vi "CodigoLabView 4_1 2024.vi"() -> (11 "Releb 2":bool)   [LabVIEW 2024]
uses:
  <vilib>/addons/_office/NI_ReportGenerationToolkit.lvlib
  <vilib>/addons/_office/excel.llb/Excel Easy Table (str).vi
  <vilib>/Utility/NIReport.llb/NI_report.lvclass
  <vilib>/Utility/NIReport.llb/Report Type.ctl
  <vilib>/Utility/NIReport.llb/NI_ReportGenerationCore.lvlib
  <vilib>/Utility/NIReport.llb/Excel/NI_Excel.lvclass
  <vilib>/Instr/_visa.llb/VISA Configure Serial Port (Instr).vi
panel:
  out "RI 4":bool
  out "RI 3":bool
  out "RI 2":bool
  out "RS 4":bool
  out "RS 3":bool
  out "RS 2":bool
  out "RS 1":bool
  out "RI 1":bool
  out "errorout":errorcluster
  out "Vrno":refnum<visa-resource-name>
  out "Texto":path=path "C:/Users/Lucas Navarro/Desktop/Ruka/ME2/pf/Jamon.txt"
  out "Historial Tensión de Línea":dbl[](graph)
  out "Historial Tomacorriente 4":dbl[](graph)
  out "Historial Tomacorriente 3":dbl[](graph)
  out "Historial Tomacorriente 2":dbl[](graph)
  out "Historial Tomacorriente 1":dbl[](graph)
  in  "?":bool
  in  "RUTA DE REGISTRO":path
  out "NP4":dbl(knob) scale=0.0..100.0
  out "NP3":dbl(knob) scale=0.0..100.0
  out "NP2":dbl(knob) scale=0.0..100.0
  out "R ON 4":bool
  out "R ON 3":bool
  out "R ON 2":bool
  out "ST":string
  out "R ON 1":bool
  out "NT":dbl(knob) scale=100.0..300.0
  out "NP1":dbl(knob) scale=0.0..100.0
  out "Releb 4":bool
  out "Relea 4":bool
  out "Rele 4":bool
  out "T4":bool
  out "Estado 4":string
  in  "Relé N°4":bool
  out "SP4":string
  out "Releb 3":bool
  out "Relea 3":bool
  out "Rele 3":bool
  out "T3":bool
  out "Estado 3":string
  out "SP3":string
  in  "Relé N°3":bool
  out "Relea 2":bool
  out "Rele 2":bool
  out "T2":bool
  out "Estado 2":string
  out "SP2":string
  in  "Relé N°2":bool
  out "Releb 1":bool
  out "Relea 1":bool
  out "Rele 1":bool
  out "T1":bool
  out "Estado 1":string
  out "SP1":string
  in  "Relé N°1":bool
  in  "PUERTO DE COMUNICACIÓN":refnum<visa-resource-name>
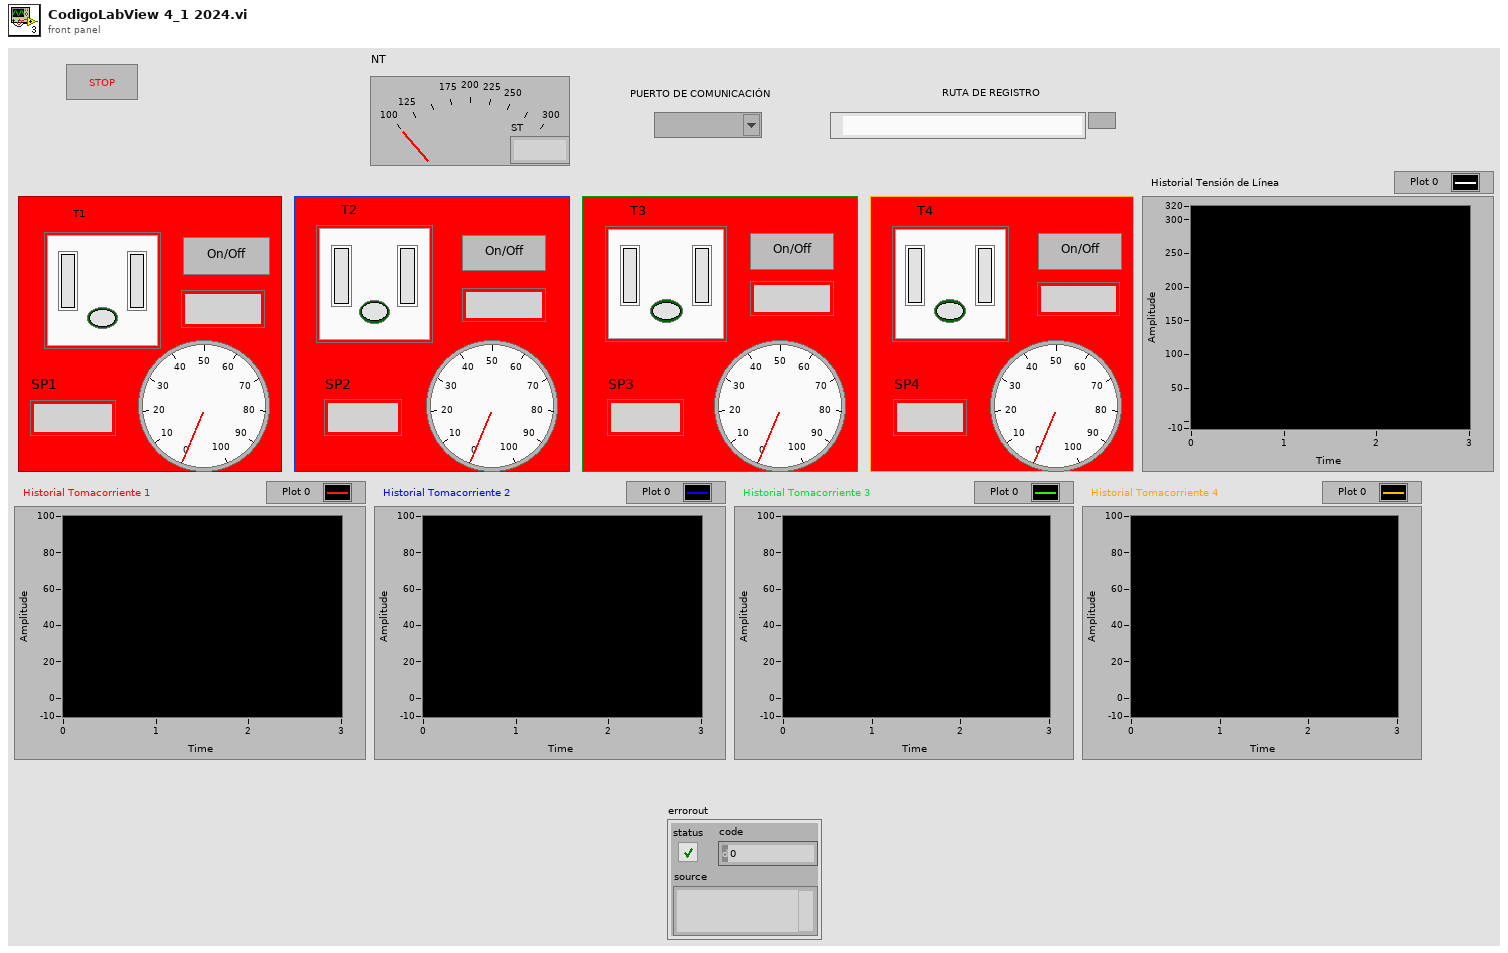
[diagram p1: front panel]
types:
  T1 = typedef "NI_ReportGenerationCore.lvlib/Report Type.ctl" = enum16{"HTML", "Word", "Excel"}
  T2 = cluster{"W1":string, "W2":string, "W3":string, "W4":string, "V":string}
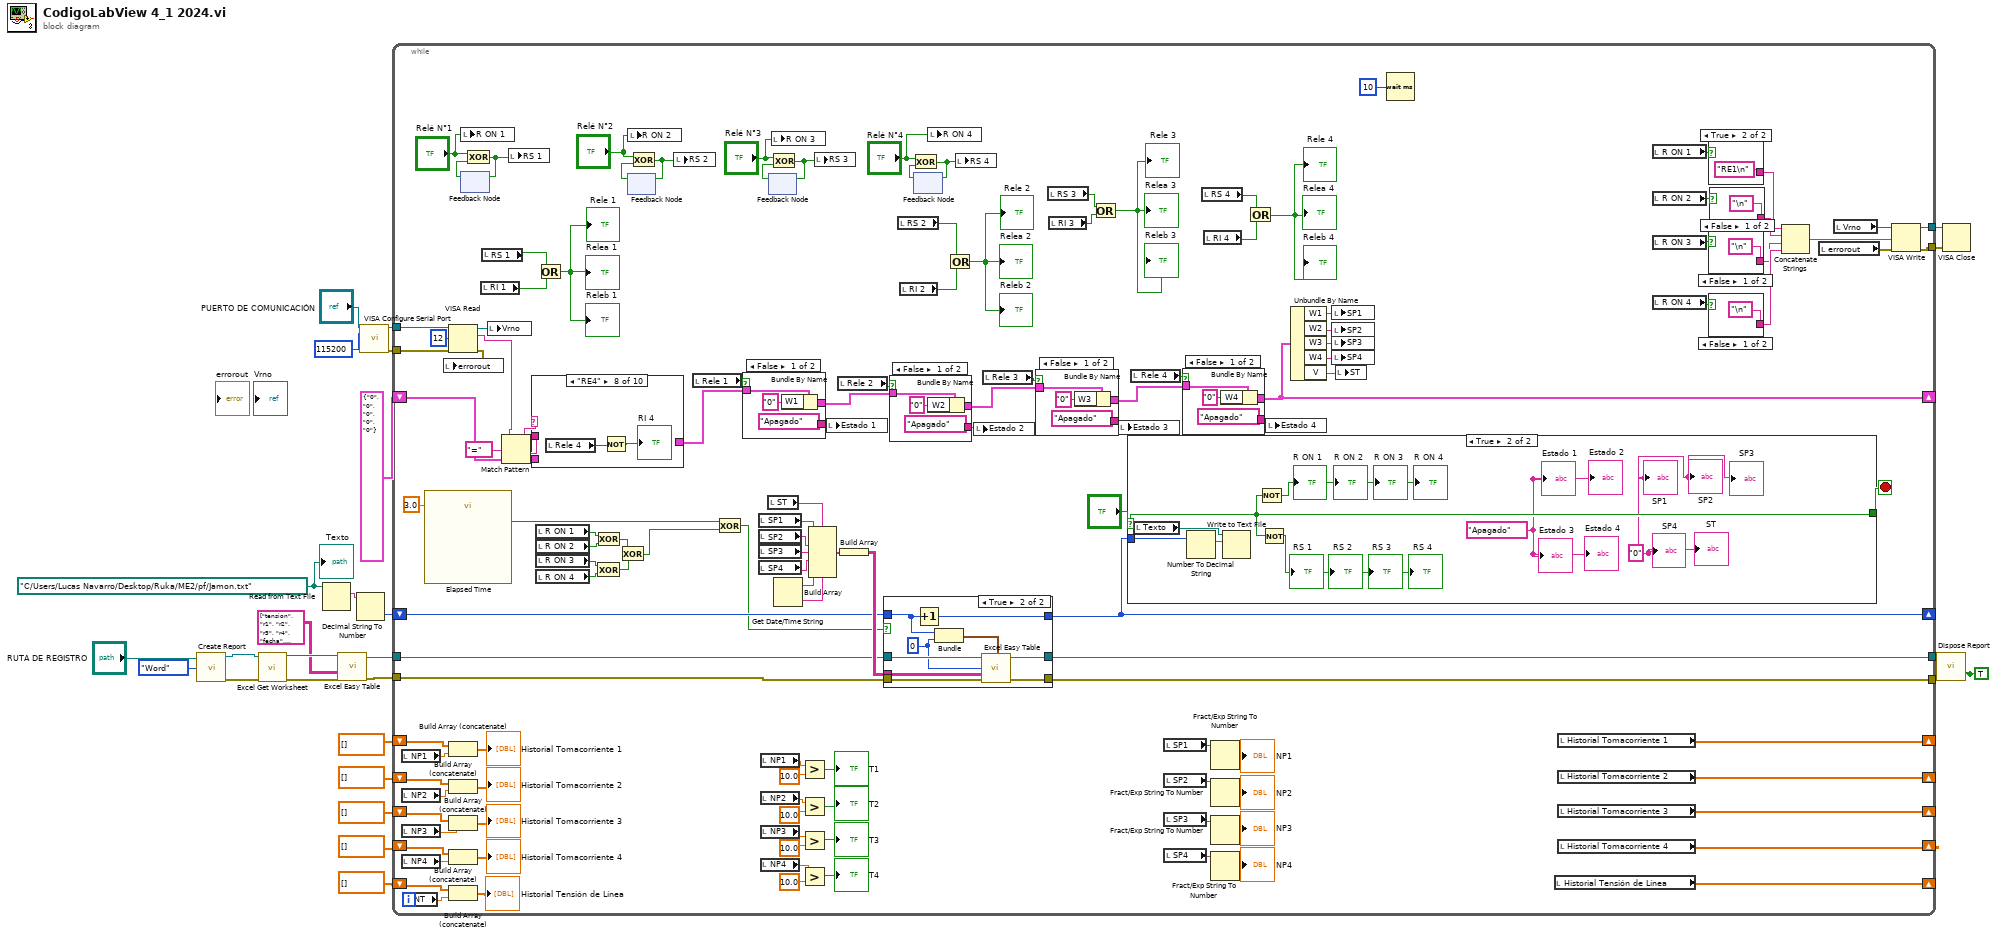
[diagram p0: block diagram]
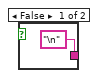
[diagram p2: hidden frame]
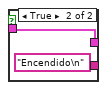
[diagram p3: hidden frame]
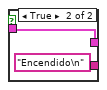
[diagram p4: hidden frame]
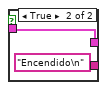
[diagram p5: hidden frame]
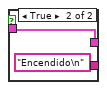
[diagram p8: hidden frame]
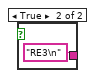
[diagram p9: hidden frame]
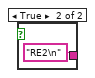
[diagram p10: hidden frame]
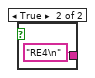
[diagram p11: hidden frame]
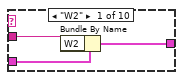
[diagram p12: hidden frame]
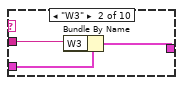
[diagram p13: hidden frame]
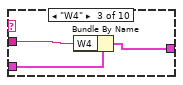
[diagram p14: hidden frame]
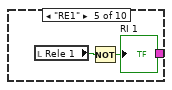
[diagram p16: hidden frame]
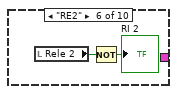
[diagram p17: hidden frame]
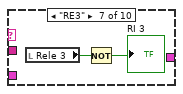
[diagram p18: hidden frame]
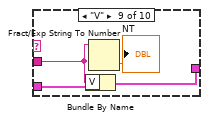
[diagram p19: hidden frame]
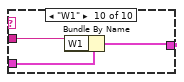
[diagram p20: hidden frame]
diagram:
  w3 = path "C:/Users/Lucas Navarro/Desktop/Ruka/ME2/pf/Jamon.txt" ("file (use dialog)")
  w2 = TRUE ("close report? (T)")
  n1 = call <vilib>:"Create Report.vi"("report type"=Report_Type."Word", "template (empty)"="RUTA DE REGISTRO") -> ("report out"=w19:refnum<class "NI_report.lvclass">, "error out"=w18:errorcluster)  [unwired: 12 in]
  n2 = call <vilib>:"Excel Get Worksheet.vi"("report in"=w19, "error in (no error)"=w18) -> ("report out"=w17:refnum<class "NI_report.lvclass">, "error out"=w16:errorcluster)  [unwired: 12 in]
  n3 = Read from Text File(file (use dialog)=w3) -> (text=w10:string)  [unwired: 3 in, 3 out]
  n4 = call-poly <vilib>:"Excel Easy Table.vi"("report in"=w17, "text data"=string[][] [["tension", "r1", "r2", "r3", "r4", "fecha", "hora"]], "error in (no error)"=w16) -> ("report out"=w14:refnum<class "NI_report.lvclass">, "error out"=w13:errorcluster)  [unwired: 8 in, 3 out]
  n5 = Decimal String To Number(string=w10) -> (number=w9:i32)  [unwired: 2 in, 1 out]
  n6 = call-poly "VISA Configure Serial Port"("VISA resource name"="PUERTO DE COMUNICACIÓN", "baud rate (9600)"=u32 115200) -> ("VISA resource name out"=w27:refnum<visa-resource-name>, "error out"=w24:errorcluster)  [unwired: 12 in]
  n7 = while {
    tunnel: w27 -> [w139]
    tunnel: w24 -> [w138]
    shift-right: [w91] -> _
    shift-left: T2 {"W1"="0", "W2"="0", "W3"="0", "W4"="0", "V"="0"} -> [w90]
    tunnel: [w141] -> w1
    tunnel: [w140] -> w22
    shift-right: [w100] -> _
    shift-left: w9 -> [w109]
    tunnel: w14 -> [w130]
    tunnel: w13 -> [w129]
    tunnel: [w122] -> w12
    tunnel: [w121] -> w11
    shift-right: [w47] -> _
    shift-left: dbl[] [] ("array") -> [w118]
    shift-right: [w48] -> _
    shift-left: dbl[] [] ("array") -> [w117]
    shift-right: [w49] -> _
    shift-left: dbl[] [] ("array") -> [w116]
    shift-right: [w51] -> _
    shift-left: dbl[] [] ("array") -> [w115]
    shift-right: [w50] -> _
    shift-left: dbl[] [] ("array") -> [w114]
    stop <- w119 stop-if-true
    n8 = local read "NP1"() -> (w73:dbl)
    n9 = local read "NP2"() -> (w72:dbl)
    n10 = local read "NP3"() -> (w71:dbl)
    n11 = local read "NP4"() -> (w70:dbl)
    n12 = local read "NT"() -> (w69:dbl)
    n13 = call "Elapsed Time"("Time Target (s)"=3.0) -> ("Time has Elapsed"=w45:bool)  [unwired: 11 in, 7 out]
    n14 = VISA Read(VISA resource name=w139, byte count=u32 12 ("Bytes at Port"), error in (no error)=w138) -> (VISA resource name out=w95:refnum<visa-resource-name>, read buffer=w89:string, error out=w94:errorcluster)  [unwired: 1 out]
    n15 = local write "errorout"(w94) -> ()
    n16 = Build Array (concatenate)(w118, w73) -> (→"Historial Tomacorriente 1":dbl[])
    n17 = Build Array (concatenate)(w117, w72) -> (→"Historial Tomacorriente 2":dbl[])
    n18 = Build Array (concatenate)(w116, w71) -> (→"Historial Tomacorriente 3":dbl[])
    n19 = Build Array (concatenate)(w115, w70) -> (→"Historial Tomacorriente 4":dbl[])
    n20 = Build Array (concatenate)(w114, w69) -> (→"Historial Tensión de Línea":dbl[])
    n21 = local write "R ON 1"("Relé N°1") -> ()
    n22 = feedback #1() -> (w157:bool)  [unwired: 1 in]
    n23 = Exclusive Or(1:w157, 2:"Relé N°1") -> (0:w99:bool)
    n24 = feedback-in #1(w99) -> ()
    n25 = local read "RI 1"() -> (w42:bool)
    n26 = local read "RS 1"() -> (w43:bool)
    n27 = local write "Vrno"(w95) -> ()
    n28 = Match Pattern(string=w89, regular expression="=") -> (before substring=w158:string, after substring=w143:string)  [unwired: 1 in, 2 out]
    n29 = local write "RS 1"(w99) -> ()
    n30 = case shown="\"RE4\"" w158 {
      tunnel: w143 -> [w213 w216 w219 _ _ _ _ _ w232 w235]
      tunnel: w90 -> [w215 w218 w221 w222 _ _ _ _ w234 w237]
      tunnel: [w214 w217 w220 w222 _ _ _ _ w233 w236] -> w137
      frame "W2" {
        n31 = Bundle By Name(cluster=w215, "W2"=w213) -> (w214:T2)
      }
      frame "W3" {
        n32 = Bundle By Name(cluster=w218, "W3"=w216) -> (w217:T2)
      }
      frame "W4" {
        n33 = Bundle By Name(cluster=w221, "W4"=w219) -> (w220:T2)
      }
      frame "False", Default {
      }
      frame "RE1" {
        n34 = local read "Rele 1"() -> (w223:bool)
        n35 = Not(x=w223) -> (.not. x?=→"RI 1":bool)
      }
      frame "RE2" {
        n36 = local read "Rele 2"() -> (w226:bool)
        n37 = Not(x=w226) -> (.not. x?=→"RI 2":bool)
      }
      frame "RE3" {
        n38 = local read "Rele 3"() -> (w227:bool)
        n39 = Not(x=w227) -> (.not. x?=→"RI 3":bool)
      }
      frame "RE4" {
        n40 = local read "Rele 4"() -> (w229:bool)
        n41 = Not(x=w229) -> (.not. x?=→"RI 4":bool)
      }
      frame "V" {
        n42 = Bundle By Name(cluster=w234, "V"=w232) -> (w233:T2)
        n43 = Fract/Exp String To Number(string=w232) -> (number=→"NT":dbl)  [unwired: 3 in, 1 out]
      }
      frame "W1" {
        n44 = Bundle By Name(cluster=w237, "W1"=w235) -> (w236:T2)
      }
    }
    n45 = local read "R ON 1"() -> (w128:bool)
    n46 = local read "R ON 2"() -> (w127:bool)
    n47 = local read "R ON 3"() -> (w125:bool)
    n48 = local read "R ON 4"() -> (w126:bool)
    n49 = Or(x=w43, y=w42) -> (x .or. y?=→"Releb 1" →"Relea 1" →"Rele 1":bool)
    n50 = Exclusive Or(1:w126, 2:w125) -> (0:w124:bool)
    n51 = Exclusive Or(1:w127, 2:w128) -> (0:w123:bool)
    n52 = Exclusive Or(1:w124, 2:w123) -> (0:w44:bool)
    n53 = local write "R ON 2"("Relé N°2") -> ()
    n54 = feedback #2() -> (w151:bool)  [unwired: 1 in]
    n55 = Exclusive Or(1:w151, 2:"Relé N°2") -> (0:w98:bool)
    n56 = feedback-in #2(w98) -> ()
    n57 = local write "RS 2"(w98) -> ()
    n58 = local read "Rele 1"() -> (w136:bool)
    n59 = Exclusive Or(1:w44, 2:w45) -> (0:w46:bool)
    n60 = case shown="False" w136 {
      tunnel: w137 -> [w203 w206]
      tunnel: [w202 w206] -> w107
      tunnel: ["Apagado" "Encendido\n"] -> w31
      frame False {
        n61 = Bundle By Name(cluster=w203, "W1"="0") -> (w202:T2)
      }
      frame True {
      }
    }
    n62 = local read "SP1"() -> (w77:string)
    n63 = local read "SP2"() -> (w76:string)
    n64 = local read "SP3"() -> (w75:string)
    n65 = local read "SP4"() -> (w74:string)
    n66 = local read "NP1"() -> (w68:dbl)
    n67 = local read "NP2"() -> (w67:dbl)
    n68 = local read "NP3"() -> (w66:dbl)
    n69 = local read "NP4"() -> (w65:dbl)
    n70 = local read "ST"() -> (w78:string)
    n71 = feedback #3() -> (w149:bool)  [unwired: 1 in]
    n72 = Exclusive Or(1:w149, 2:"Relé N°3") -> (0:w97:bool)
    n73 = feedback-in #3(w97) -> ()
    n74 = local write "R ON 3"("Relé N°3") -> ()
    n75 = Get Date/Time String() -> (date string=w134:string, time string=w135:string)  [unwired: 3 in]
    n76 = Greater?(x=w68, y=10.0) -> (0:→"T1":bool)
    n77 = Greater?(x=w67, y=10.0) -> (0:→"T2":bool)
    n78 = Greater?(x=w66, y=10.0) -> (0:→"T3":bool)
    n79 = Greater?(x=w65, y=10.0) -> (0:→"T4":bool)
    n80 = Build Array(w78, w77, w76, w75, w74, w134, w135) -> (w132:string[])
    n81 = local write "RS 3"(w97) -> ()
    n82 = local write "Estado 1"(w31) -> ()
    n83 = local read "Rele 2"() -> (w104:bool)
    n84 = Build Array(w132) -> (w133:string[][])
    n85 = case shown="True" w46 {
      tunnel: w133 -> [_ w200]
      tunnel: w129 -> [w191 w199]
      tunnel: [w190 w198] -> w122
      tunnel: [w191 w197] -> w121
      tunnel: w130 -> [w190 w196]
      tunnel: w109 -> [w189 w195]
      tunnel: [w189 w194] -> w100
      frame False {
      }
      frame True {
        w192 = 0 ("iteration")
        n86 = Increment(x=w195) -> (x+1=w194:i32)
        n87 = Bundle(w195, "iteration"=w192) -> (w193:cluster{i32, "iteration":i32})  [unwired: 1 in]
        n88 = call-poly <vilib>:"Excel Easy Table.vi"("report in"=w196, "iteration"=w192, "start (0, 0)"=w193, "text data"=w200, "error in (no error)"=w199) -> ("report out"=w198:refnum<class "NI_report.lvclass">, "error out"=w197:errorcluster)  [unwired: 6 in, 3 out]
      }
    }
    n89 = case shown="False" w104 {
      tunnel: w107 -> [w177 w180]
      tunnel: [w176 w180] -> w106
      tunnel: ["Apagado" "Encendido\n"] -> w30
      frame False {
        n90 = Bundle By Name(cluster=w177, "W2"="0") -> (w176:T2)
      }
      frame True {
      }
    }
    n91 = local read "RS 2"() -> (w40:bool)
    n92 = local read "RI 2"() -> (w39:bool)
    n93 = feedback #4() -> (w147:bool)  [unwired: 1 in]
    n94 = Exclusive Or(1:w147, 2:"Relé N°4") -> (0:w96:bool)
    n95 = feedback-in #4(w96) -> ()
    n96 = local write "R ON 4"("Relé N°4") -> ()
    n97 = Or(x=w40, y=w39) -> (x .or. y?=→"Releb 2" →"Relea 2" →"Rele 2":bool)
    n98 = local write "RS 4"(w96) -> ()
    n99 = local write "Estado 2"(w30) -> ()
    n100 = local read "Rele 3"() -> (w103:bool)
    n101 = case shown="False" w103 {
      tunnel: w106 -> [w171 w174]
      tunnel: [w170 w174] -> w105
      tunnel: ["Apagado" "Encendido\n"] -> w28
      frame False {
        n102 = Bundle By Name(cluster=w171, "W3"="0") -> (w170:T2)
      }
      frame True {
      }
    }
    n103 = local read "RS 3"() -> (w37:bool)
    n104 = local read "RI 3"() -> (w36:bool)
    n105 = Or(x=w37, y=w36) -> (x .or. y?=→"Relea 3" →"Releb 3" →"Rele 3":bool)
    n106 = local write "Estado 3"(w28) -> ()
    n107 = case shown="True" "?" {
      selector: "?" -> [_ w185]
      tunnel: w100 -> [_ w188]
      tunnel: [_ w185] -> w119
      frame False {
      }
      frame True {
        w181 = "0"
        w182 = "Apagado"
        n108 = local read "Texto"() -> (w186:path)
        n109 = Number To Decimal String(number=w188) -> (decimal integer string=w187:string)  [unwired: 1 in]
        n110 = Write to Text File(file (use dialog)=w186, text=w187) -> ()  [unwired: 2 in, 3 out]
        n111 = Not(x=w185) -> (.not. x?=→"R ON 1" →"R ON 2" →"R ON 3" →"R ON 4":bool)
        n112 = Not(x=w185) -> (.not. x?=→"RS 4" →"RS 3" →"RS 1" →"RS 2":bool)
        "Estado 1" <- w182
        "Estado 2" <- w182
        "Estado 3" <- w182
        "Estado 4" <- w182
        "SP1" <- w181
        "ST" <- w181
        "SP2" <- w181
        "SP3" <- w181
        "SP4" <- w181
      }
    }
    n113 = local read "Rele 4"() -> (w102:bool)
    n114 = local read "SP1"() -> (w82:string)
    n115 = local read "SP2"() -> (w80:string)
    n116 = local read "SP3"() -> (w79:string)
    n117 = local read "SP4"() -> (w81:string)
    n118 = case shown="False" w102 {
      tunnel: w105 -> [w165 w168]
      tunnel: [w164 w168] -> w91
      tunnel: ["Apagado" "Encendido\n"] -> w29
      frame False {
        n119 = Bundle By Name(cluster=w165, "W4"="0") -> (w164:T2)
      }
      frame True {
      }
    }
    n120 = local read "RS 4"() -> (w33:bool)
    n121 = local read "RI 4"() -> (w34:bool)
    n122 = Fract/Exp String To Number(string=w82) -> (number=→"NP1":dbl)  [unwired: 3 in, 1 out]
    n123 = Fract/Exp String To Number(string=w80) -> (number=→"NP2":dbl)  [unwired: 3 in, 1 out]
    n124 = Fract/Exp String To Number(string=w79) -> (number=→"NP3":dbl)  [unwired: 3 in, 1 out]
    n125 = Fract/Exp String To Number(string=w81) -> (number=→"NP4":dbl)  [unwired: 3 in, 1 out]
    n126 = Or(x=w33, y=w34) -> (x .or. y?=→"Relea 4" →"Releb 4" →"Rele 4":bool)
    n127 = local write "Estado 4"(w29) -> ()
    n128 = Unbundle By Name(w91) -> ("W1"=w113:string, "W2"=w110:string, "W3"=w111:string, "W4"=w112:string, "V"=w108:string)
    n129 = local write "SP1"(w113) -> ()
    n130 = local write "SP2"(w110) -> ()
    n131 = local write "SP3"(w111) -> ()
    n132 = local write "SP4"(w112) -> ()
    n133 = local write "ST"(w108) -> ()
    n134 = Wait (ms)(milliseconds to wait=u32 10) -> ()  [unwired: 1 out]
    n135 = local read "Historial Tensión de Línea"() -> (w50:dbl[])
    n136 = local read "Historial Tomacorriente 1"() -> (w47:dbl[])
    n137 = local read "Historial Tomacorriente 2"() -> (w48:dbl[])
    n138 = local read "Historial Tomacorriente 3"() -> (w49:dbl[])
    n139 = local read "Historial Tomacorriente 4"() -> (w51:dbl[])
    n140 = local read "R ON 1"() -> (w84:bool)
    n141 = local read "R ON 2"() -> (w154:bool)
    n142 = local read "R ON 3"() -> (w153:bool)
    n143 = local read "R ON 4"() -> (w155:bool)
    n144 = case shown="True" w84 {
      tunnel: ["\n" "RE1\n"] -> w83
      frame False {
      }
      frame True {
      }
    }
    n145 = case shown="False" w153 {
      tunnel: ["\n" "RE3\n"] -> w144
      frame False {
      }
      frame True {
      }
    }
    n146 = case shown="False" w155 {
      tunnel: ["\n" "RE4\n"] -> w145
      frame False {
      }
      frame True {
      }
    }
    n147 = case shown="False" w154 {
      tunnel: ["\n" "RE2\n"] -> w146
      frame False {
      }
      frame True {
      }
    }
    n148 = Concatenate Strings(w83, w146, w144, w145) -> (w142:string)
    n149 = local read "errorout"() -> (w93:errorcluster)
    n150 = local read "Vrno"() -> (w92:refnum<visa-resource-name>)
    n151 = VISA Write(VISA resource name=w92, write buffer=w142, error in (no error)=w93) -> (VISA resource name out=w141:refnum<visa-resource-name>, error out=w140:errorcluster)  [unwired: 1 out]
  }
  n152 = call-dynamic "Dispose Report.vi"("report in"=w12, "save changes? (F)"=w2, "error in (no error)"=w11, "close report? (T)"=w2) -> ()  [unwired: 11 in, 1 out]
  n153 = VISA Close(VISA resource name=w1, error in (no error)=w22) -> ()  [unwired: 1 out]
  "Texto" <- w3
